vi "Set Universal Timeout.vi"(8 "error in (no error)":errorcluster, 10 "timeout_ms (10000)":i32=10000, 11 "LabVIEWHTTPClient_NET in":refnum<class "HttpClient_NET.lvclass">) -> (0 "error out":errorcluster, 3 "LabVIEWHTTPClient_NET out":refnum<class "HttpClient_NET.lvclass">)   [LabVIEW 2018, in "HttpClient_NET.lvlib" / "HttpClient_NET.lvclass"]
doc: "<b> </b> <b> </b>\nHttpClient_NET\nJustin Young - Viviota\nCopyright (c) 2021\nLicense: BSD"
uses:
  HttpClient_NET.lvclass
  HttpClient_NET.lvclass/HttpClient_NET.ctl
  Accessors/Read NET_HttpClient.vi
  System.Net.Http
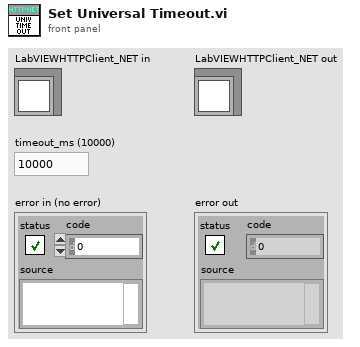
[diagram p1: front panel]
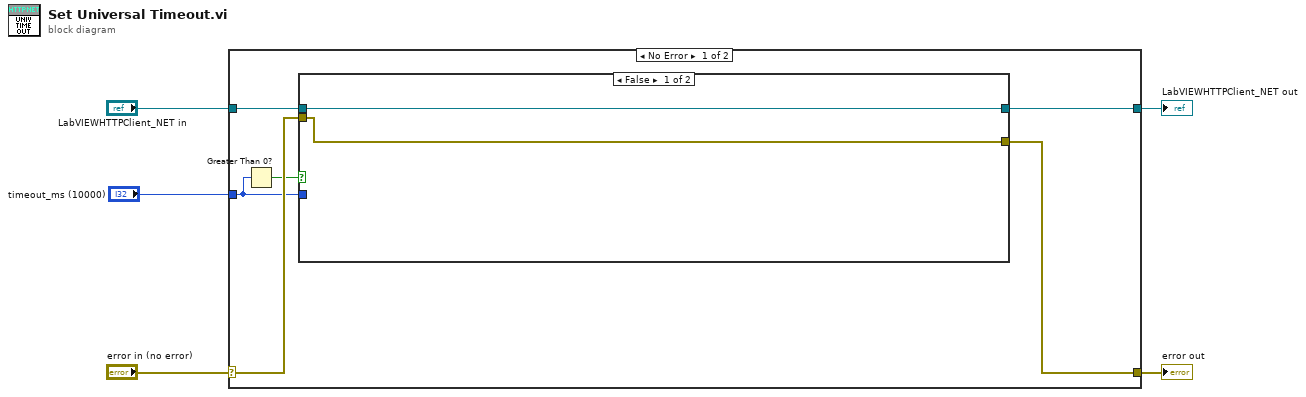
[diagram p0: block diagram]
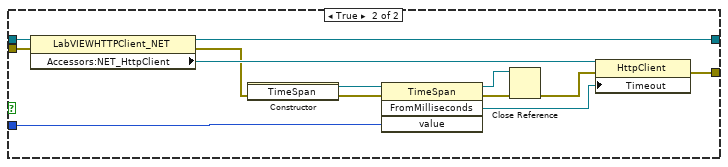
[diagram p2: hidden frame]
diagram:
  n1 = case shown="No Error" "error in (no error)" {
    selector: "error in (no error)" -> [w9 w28]
    tunnel: [w8 w28] -> w4
    tunnel: [w10 w27] -> w2
    tunnel: "LabVIEWHTTPClient_NET in" -> [w11 w27]
    tunnel: "timeout_ms (10000)" -> [w7 _]
    frame No Error {
      n2 = Greater Than 0?(x=w7) -> (x > 0?=w6:bool)
      n3 = case shown="False" w6 {
        tunnel: w11 -> [w13 w26]
        tunnel: [w13 w25] -> w10
        tunnel: w9 -> [w12 w23]
        tunnel: [w12 w20] -> w8
        tunnel: w7 -> [_ w14]
        frame False {
        }
        frame True {
          n4 = property class="LabVIEWHTTPClient_NET"(reference=w26, error in=w23) -> (reference out=w25:refnum<class "HttpClient_NET.lvclass">, error out=w22:errorcluster, "Accessors:NET_HttpClient"=w24:refnum<k24>)
          n5 = constructor class="TimeSpan"(error in=w22) -> (reference out=w18:refnum<k24>, error out=w21:errorcluster)  [unwired: 2 in, 1 out]
          n6 = invoke class="TimeSpan" method="FromMilliseconds"(reference=w18, error in=w21, "value"=w14) -> (reference out=w15:refnum<k24>, error out=w19:errorcluster, "FromMilliseconds"=w17:refnum<k24>)  [unwired: 1 in, 1 out]
          n7 = Close Reference(reference=w15, error in (no error)=w19) -> (error out=w16:errorcluster)
          n8 = property class="HttpClient"(reference=w24, error in=w16, "Timeout"=w17) -> (error out=w20:errorcluster)  [unwired: 1 out]
        }
      }
    }
    frame Error {
    }
  }
  "error out" <- w4
  "LabVIEWHTTPClient_NET out" <- w2
